vi "Reverse 2D Array.vi"(1 "Rev. Columns":bool, 2 "Input array":dbl[][](array[numeric]) format="%.2e") -> (0 "Output Array":dbl[][](array[numeric]) format="%.2e")   [LabVIEW 2021]
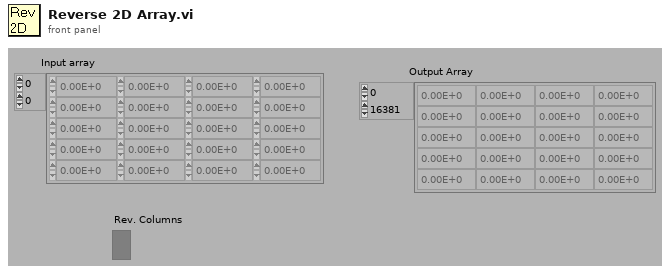
[diagram p1: front panel]
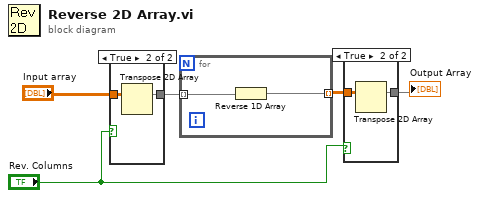
[diagram p0: block diagram]
diagram:
  n1 = case shown="True" "Rev. Columns" {
    tunnel: [w6 w8] -> w5
    tunnel: "Input array" -> [w6 w7]
    frame False {
    }
    frame True {
      n2 = Transpose 2D Array(2D array=w7) -> (transposed array=w8:dbl[][])
    }
  }
  n3 = for {
    tunnel: w5 -> [w10] mode=indexing
    tunnel: [w9] -> w4 mode=indexing
    n4 = Reverse 1D Array(array=w10) -> (reversed array=w9:dbl[])
  }
  n5 = case shown="True" "Rev. Columns" {
    tunnel: [w11 w13] -> w3
    tunnel: w4 -> [w11 w12]
    frame False {
    }
    frame True {
      n6 = Transpose 2D Array(2D array=w12) -> (transposed array=w13:dbl[][])
    }
  }
  "Output Array" <- w3
